vi "Build Package Path.vi"(0 "Project Path":path, 11 "error in (no error)":errorcluster) -> (4 "Package Directory":path, 15 "error out":errorcluster)   [LabVIEW 2021, in "Measurement Builder.lvlib"]
uses:
  Measurement Builder.lvlib
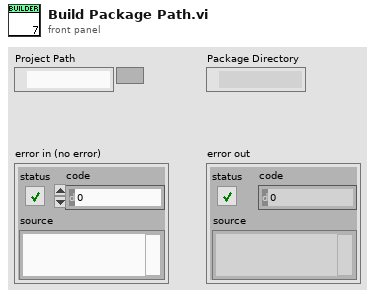
[diagram p1: front panel]
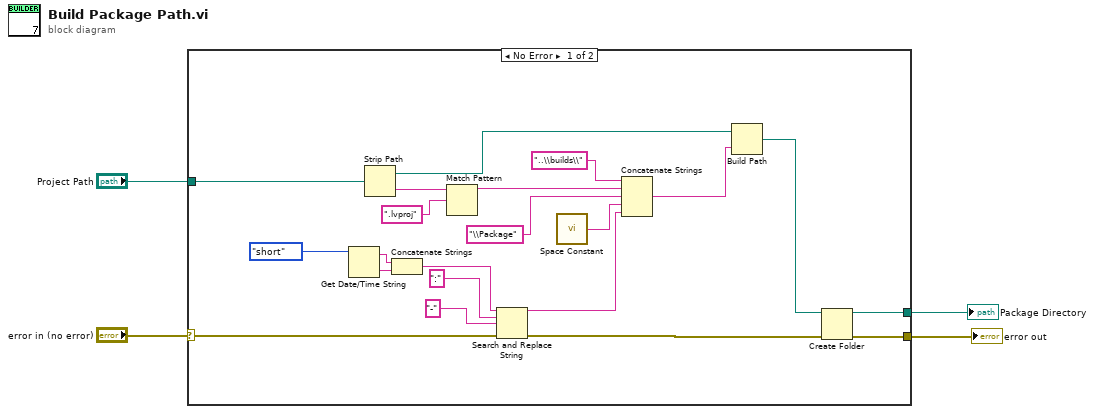
[diagram p0: block diagram]
diagram:
  n1 = case shown="No Error" "error in (no error)" {
    selector: "error in (no error)" -> [w5 w26]
    tunnel: "Project Path" -> [w17 _]
    tunnel: [w13 _] -> w3
    tunnel: [w6 w26] -> w2
    frame No Error {
      n2 = Get Date/Time String(date format (0)=enum16{"short", "long", "abbreviated"}."short") -> (date string=w20:string, time string=w21:string)  [unwired: 2 in]
      n3 = Strip Path(path=w17) -> (stripped path=w12:path, name=w9:string)
      n4 = Concatenate Strings(w20, w21) -> (w22:string)
      n5 = Match Pattern(string=w9, regular expression=".lvproj") -> (before substring=w8:string)  [unwired: 1 in, 3 out]
      n6 = Search and Replace String(input string=w22, search string=":", replace string="-" ("replace string (\"\")"), error in=w5) -> (result string=w16:string, error out=w7:errorcluster)  [unwired: 4 in, 2 out]
      n7 = call <vilib>:"Space Constant.vi"() -> ("String"=w11:string)
      n8 = Concatenate Strings("..\\builds\\" ("string"), w8, "\\Package" ("string"), w11, w16) -> (w15:string)
      n9 = Build Path(base path=w12, name or relative path=w15) -> (appended path=w14:path)
      n10 = Create Folder(path (use dialog)=w14, error in=w7) -> (created path=w13:path, error out=w6:errorcluster)  [unwired: 1 in, 1 out]
    }
    frame Error {
    }
  }
  "Package Directory" <- w3
  "error out" <- w2
